vi "(Old Driver) Block Read Iterator.vi"(8 "error in (no error)":errorcluster, 9 "Iterations (1000)":i32=110, 10 "Channel Count":i32, 11 "VMIC-5565":T1) -> (0 "error out":errorcluster, 1 "Histogram Graph":T2(graph), 2 "Metrics":T3 {"Transfer Rate" format="%.2pB/s"; "Duration Std. Dev." format="%.0f µs"; "Duration Average" format="%.0f µs"}, 3 "VMIC-5565 out":T1)   [LabVIEW 2016]
uses:
  Controls/Throughput Metrics.ctl
  <instrlib>/GE 5565 PIORC/Public/DMA Interrupt/GE5565 DMA Read Interrupt (U8) Cluster.vi
  <instrlib>/GE 5565 PIORC/GE 5565 PIORC.lvlib
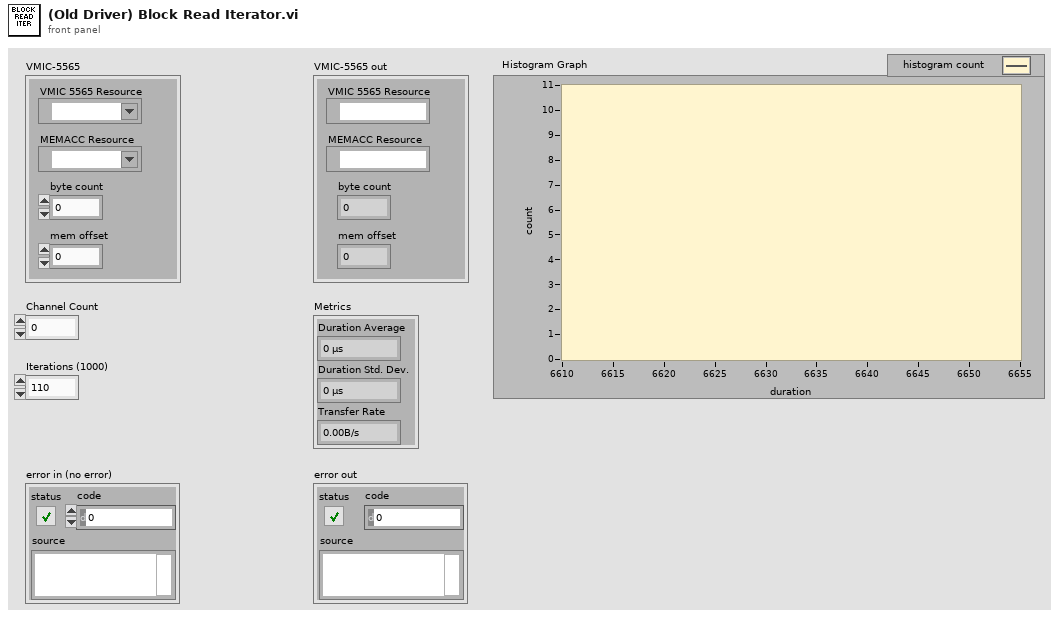
[diagram p1: front panel]
types:
  T1 = cluster{"VMIC 5565 Resource":refnum<visa-resource-name>, "MEMACC Resource":refnum<visa-resource-name>, "byte count":u32, "mem offset":u32}
  T2 = cluster{"X Values":dbl[], "Histogram: h(x)":i32[]}
  T3 = typedef "Throughput Metrics.ctl" = cluster{"Duration Average":u32, "Duration Std. Dev.":u32, "Transfer Rate":dbl}
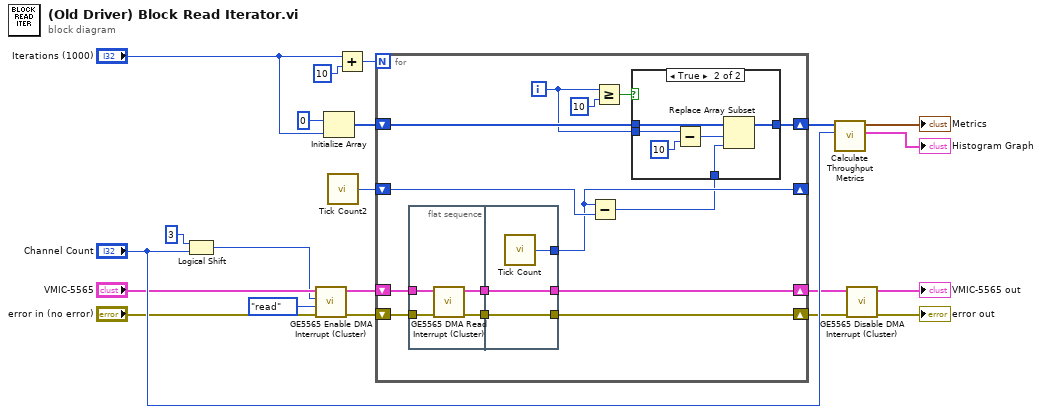
[diagram p0: block diagram]
diagram:
  n1 = Logical Shift(y=i16 3, x="Channel Count") -> (x << y=w6:i32)
  n2 = call <instrlib>:"GE5565 Enable DMA Interrupt (Cluster).vi"("error in (no error)"="error in (no error)", "operation (read)"=enum16{"read", "write"}."read", "transfer size (1024 bytes)"=w6, "VMIC reference in"="VMIC-5565") -> ("error out"=w9:errorcluster, "VMIC reference out"=w10:T1)  [unwired: 2 in]
  n3 = Initialize Array(u32 0 ("x-y"), "Iterations (1000)") -> (w15:u32[])
  n4 = call "Tick Count2"() -> ("Tick Count(uSec)"=w19:u32)
  n5 = Add(x="Iterations (1000)", y=10) -> (x+y=w21:i32)
  n6 = for {
    N: w21 -> [_]
    shift-right: [w27] -> _
    shift-left: w19 -> [w28]
    shift-right: [w30] -> w4
    shift-left: w10 -> [w35]
    shift-right: [w29] -> w3
    shift-left: w9 -> [w34]
    shift-right: [w25] -> w14
    shift-left: w15 -> [w26]
    i -> [w23]
    n7 = flat-sequence {
      tunnel: w35 -> [w46]
      tunnel: w34 -> [w45]
      tunnel: [w44] -> w33
      tunnel: [w43] -> w32
      tunnel: [w49] -> w30
      tunnel: w33 -> [w49]
      tunnel: w32 -> [w48]
      tunnel: [w48] -> w29
      tunnel: [w47] -> w27
      frame #0 {
        n8 = call-poly <instrlib>:"GE5565 DMA Read Interrupt (Cluster).vi"("error in (no error)"=w45, "VMIC reference in"=w46) -> ("error out"=w43:errorcluster, "VMIC reference out"=w44:T1)  [unwired: 7 in, 1 out]
      }
      frame #1 {
        n9 = call "Tick Count"() -> ("Tick Count(uSec)"=w47:u32)
      }
    }
    n10 = Subtract(x=w27, y=w28) -> (x-y=w22:u32)
    n11 = Greater Or Equal?(x=w23, y=10) -> (x >= y?=w24:bool)
    n12 = case shown="True" w24 {
      tunnel: w26 -> [w36 w42]
      tunnel: [w36 w41] -> w25
      tunnel: w23 -> [_ w40]
      tunnel: w22 -> [_ w37]
      frame False {
      }
      frame True {
        n13 = Subtract(x=w40, y=10) -> (x-y=w38:i32)
        n14 = Replace Array Subset(array=w42, new element=w37, index=w38) -> (w41:u32[])
      }
    }
  }
  n15 = call "Calculate Throughput Metrics.vi"("Channel Count"="Channel Count", "Durations"=w14) -> ("Histogram Graph"=→"Histogram Graph":T2, "Metrics"=→"Metrics":T3)  [unwired: 8 in]
  n16 = call <instrlib>:"GE5565 Disable DMA Interrupt (Cluster).vi"("error in (no error)"=w3, "VMIC reference in"=w4) -> ("error out"=→"error out":errorcluster, "VMIC reference out"=→"VMIC-5565 out":T1)  [unwired: 4 in]
